vi "Day 2 task 2.vi"() -> ()   [LabVIEW 2022 SP3]
uses:
  <vilib>/regexp/Match Regular Expression.xnode
panel:
  out "sum":i32
  out "Array":i32[](array[numeric])
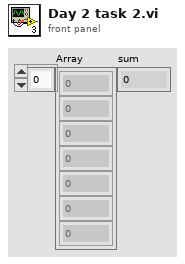
[diagram p1: front panel]
types:
  T1 = cluster{"Their":string, "Win":string, "Loose":string}[]
  T2 = cluster{"Mine":string, "Theirs":string, "Score":i32}[]
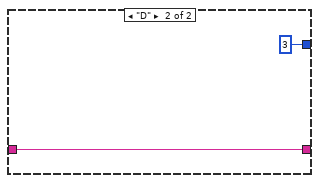
[diagram p2: hidden frame]
diagram:
  (unwired) "A Y\nB X\nC Z"
  (unwired) T2 [{"Mine"="R", "Theirs"="P", "Score"=0}, {"Mine"="R", "Theirs"="S", "Score"=6}, {"Mine"="P", "Theirs"="R", "Score"=6}, {"Mine"="P", "Theirs"="S", "Score"=0}, {"Mine"="S", "Theirs"="R", "Score"=0}, {"Mine"="S", "Theirs"="P", "Score"=6}]
  w9 = TRUE ("replace all? (F)")
  n1 = Search and Replace String(replace all?=w9, input string="C Y\nC Y\nB Y\nA Z\nB Z\nA X\nA Y\nA Y\nA X\nA Y\nB Y\nA Y\nB Y\nB Y\nB Z\nB Z\nB Z\nB Z\nA Y\nB Z\nA Y\nB X\nB Y\nB X\nA X\nA X\nB Z\nA X\nA X\nB Z\nB Z\nB Y\nB Z\nB Z\nB Z\nB Y\nA X\nA X\nB Z\nA X\nB X\nB X\nC Y\nB Z\nC X\nA X\nA Y\nB Y\nA Y\nB X\nA X\nB Y\nB Z\nB Z\nB Y\nB Z\nC Z\nB X\nB X\nB Z\nB Z\nB Z\nB Z\nA Y\nB X\nA X\nC X\nB Y\nB Z\nA Y\nB Z\nB Z\nB Y\nB Y\nB Z\nB Y\nB Z\nA X\nB X\nB X\nA X\nA X\nB Z\nB Z\nB Z\nB Z\nB Y\nB X\nB Z\nA X\nA Y\nB Z\nA Y\nB Z\nB Y\nB Z\nA X\nB Y\nA Y\nB Z\nA Z\nA Y\nA Y\nC Y\nB Z\nB X\nA Z\nB Z\nA X\nB Z\nA Z\nB Z\nA X\nB Y\nA X\nB Y\nB Z\nB X\nB X\nB Z\nB Z\nB Z\nA X\nB Z\nA X\nB X\nB Z\nA X\nC Z\nB Z\nB Z\nB Y\nB Y\nB Y\nB Z\nB Z\nA Y\nB Z\nB Z\nC Y\nC Z\nA X\nB Z\nB X\nB Z\nB Z\nB Y\nA X\nB Z\nB Y\nA Z\nB Z\nA X\nA X\nB Y\nA Y\nB Z\nB Z\nB X\nB Y\nA X\nA Y\nB X\nC Z\nA Y\nB Z\nB Z\nB Z\nA Z\nC Y\nB Y\nB Y\nB Z\nC Y\nB Y\nB X\nB X\nB Z\nC Z\nA X\nB Z\nB Z\nB Z\nB Z\nB X\nB X\nA X\nA Z\nA Z\nA X\nC Y\nB X\nA X\nA Y\nA X\nB X\nA Y\nB Z\nB Z\nA Y\nA X\nB Y\nB Z\nB Z\nA X\nA Z\nB Z\nB X\nA X\nB Z\nB Y\nA Y\nA Z\nB X\nA Y\nB Z\nA Z\nB Z\nA Y\nB Z\nB X\nB Y\nA Y\nB Z\nB Z\nA X\nA X\nB Y\nB Z\nA X\nB Z\nB Z\nB Z\nB Z\nB Z\nA Z\nB Z\nB Z\nB X\nA Y\nC X\nB Z\nB Y\nB Y\nB Z\nB Z\nB Z\nB Y\nB X\nB Y\nC X\nB Z\nA Z\nA Y\nC X\nA X\nB X\nA X\nB X\nA Y\nB Z\nA Y\nA Y\nB Z\nB X\nB Z\nA Y\nB Z\nB X\nC Z\nC X\nC Z\nB Y\nB X\nB Z\nB Z\nB Y\nB Z\nB Y\nB Z\nA X\nB X\nB Z\nA X\nB Z\nB Y\nB Z\nA X\nB Y\nC Y\nA Z\nB Z\nC Z\nA Y\nB Z\nA Y\nA Z\nB Y\nA X\nA X\nB Z\nB Z\nB Z\nA Y\nB Z\nA Z\nB Z\nA Y\nA Z\nB Y\nC Z\nB Z\nA Z\nB X\nB Z\nB Y\nB Z\nA Z\nA Z\nB Z\nB X\nC Z\nB X\nB Z\nB Y\nA X\nB Z\nA X\nB X\nB Z\nB Z\nA X\nB X\nC X\nC X\nB X\nB Y\nB Z\nB X\nB Y\nB Y\nB Z\nA Z\nB Z\nC X\nA Y\nC X\nB Z\nA Y\nB Z\nB Y\nB Z\nB X\nA X\nB X\nB Z\nA Y\nA Y\nB Z\nB Z\nB Z\nA Y\nB Z\nB X\nC X\nB Z\nB Z\nC Y\nB Z\nC Y\nB Z\nC Y\nC X\nB Z\nC Y\nA Y\nA Y\nC Z\nB Z\nB X\nB Z\nB X\nC Z\nB Z\nA Z\nB Z\nC Y\nB Z\nA X\nA Y\nB Y\nB Y\nB Z\nA Y\nB X\nB Z\nB Z\nA Z\nB X\nA Y\nA Y\nB Z\nB Z\nB Z\nC X\nA Z\nB X\nC Z\nB Y\nB Z\nB X\nA Y\nB Z\nA X\nB X\nB Y\nA Y\nB Z\nB Z\nB Y\nA Z\nB Z\nA X\nB Y\nA Y\nA X\nA Y\nA X\nA X\nB X\nB Y\nB X\nB Y\nB Z\nB Y\nB X\nA X\nB Z\nA Z\nA X\nB Z\nB Y\nA X\nB Y\nA X\nB X\nC Y\nB X\nB X\nB X\nC Y\nB X\nB Y\nB Y\nB Y\nB Y\nB X\nA Y\nC Y\nB Z\nB Z\nB X\nB Z\nC Y\nB Y\nB Z\nB Z\nB Y\nB Z\nA X\nB X\nB Y\nA X\nC Y\nB Z\nA Y\nB Z\nB Z\nB Z\nA X\nB Y\nB Z\nB Y\nB Z\nA X\nB Z\nA X\nB Y\nB Y\nB X\nB X\nA Y\nB Z\nC Y\nA X\nA X\nB X\nB Z\nB X\nB X\nB Z\nB Z\nA X\nB X\nB Z\nA Z\nB Y\nA X\nB Z\nC Y\nB Z\nB X\nB Z\nB Z\nA Y\nA Y\nB Z\nB X\nB Y\nB Z\nA Y\nA Y\nB X\nB X\nC X\nB Z\nC Z\nB X\nA Y\nB Z\nA Z\nB Y\nA Y\nB Z\nB X\nB X\nA Y\nB Z\nB Y\nA X\nB Y\nB Y\nB Y\nB X\nB Y\nB Z\nB Y\nB Y\nA X\nC Z\nB Z\nB Z\nA Z\nB Z\nB Z\nA X\nB X\nA Y\nA X\nB X\nC X\nB X\nB Z\nB Y\nA Z\nA Y\nB Y\nB Z\nB X\nB X\nB Z\nB Z\nB Y\nA X\nB Z\nA Y\nA X\nB Y\nB Z\nB Z\nB X\nA X\nA Y\nC X\nA Y\nB Z\nB Y\nB Z\nB Z\nC Z\nB Z\nB X\nA X\nC Y\nB X\nB Z\nA Z\nA X\nA Y\nB Z\nB Z\nA Y\nA Y\nB X\nA Y\nA Y\nB Z\nA Y\nB Y\nB Z\nA Y\nA Z\nB X\nB X\nB Y\nB Z\nB Z\nA X\nB X\nC X\nB Y\nA Y\nA X\nA X\nA X\nB Y\nA X\nA Z\nA Y\nB X\nA Y\nB Z\nC X\nB X\nB X\nB Z\nB X\nB X\nB Z\nA X\nB Z\nB X\nB Z\nA Y\nB Y\nB Z\nB Y\nB Z\nB Z\nA X\nB Z\nA Y\nC Z\nA Y\nB Z\nA Y\nB X\nB Z\nB X\nC Y\nA X\nB Z\nB Y\nA X\nA X\nB X\nB Z\nA Z\nB Z\nB X\nB X\nB X\nB Z\nB Z\nB Y\nB X\nB X\nA X\nB Z\nB X\nA X\nA X\nA X\nB X\nB Z\nA Z\nB X\nB Y\nB Y\nB Z\nB Z\nC Z\nA Y\nA X\nB Y\nB X\nB Z\nB X\nA X\nB Z\nB Z\nB Y\nB Z\nB X\nB Z\nB Z\nB X\nB X\nA X\nA X\nB X\nB Z\nB Z\nC X\nC X\nB Z\nB Z\nB X\nB Z\nB Y\nB X\nA X\nB Y\nA Y\nA X\nB Z\nB Z\nC X\nB Y\nB Z\nB Z\nB X\nB Z\nB Z\nC Z\nB Z\nB Y\nB Z\nB X\nA X\nB X\nB Z\nB Z\nA Y\nB Z\nB Z\nB Z\nB Z\nA X\nB Z\nB Z\nB X\nB Y\nB Y\nB Z\nA X\nB Z\nB Y\nB X\nA X\nB X\nB Z\nB Z\nB Z\nB X\nB Z\nB Z\nB Z\nA Y\nB Z\nC X\nB Y\nB Y\nB Y\nA Y\nB Z\nB Z\nA X\nC Z\nB Z\nB Z\nB Z\nB X\nB Z\nA Z\nB Z\nB Z\nB Z\nA Z\nB Z\nC Y\nB X\nA X\nA Y\nB Z\nB Z\nA Z\nB Z\nB X\nA Z\nB Y\nB Z\nB X\nB Z\nB X\nB Y\nB Z\nA X\nB Z\nB Z\nA Y\nB X\nB X\nB X\nA Z\nC X\nA Z\nB Z\nB Z\nB Z\nB X\nA Y\nC X\nA Z\nA Y\nB X\nB Z\nB X\nB Z\nB Y\nA Y\nB X\nC X\nA Y\nC Z\nA X\nB Z\nB Z\nA Z\nB X\nB Y\nB Z\nA Y\nB Y\nA X\nA X\nC Y\nA Y\nB X\nA X\nB Y\nB X\nB Y\nA Y\nA X\nC Y\nB Y\nB Y\nB Z\nB Y\nB X\nB Z\nB Z\nB X\nA X\nB Z\nB Z\nB Z\nB X\nB Z\nB X\nB Z\nB Z\nB Y\nB Y\nB X\nA X\nB Z\nB Y\nA Y\nB Z\nB X\nB Z\nB Z\nA Z\nB Z\nA Y\nB Z\nA X\nB Z\nB Z\nA Y\nB Z\nA X\nB Z\nA Y\nA Y\nA Z\nB X\nB Z\nB Y\nA Z\nC Z\nB Z\nA X\nA X\nB X\nA Z\nB X\nB X\nB Z\nC X\nB Z\nB Z\nB Z\nB Z\nB X\nA Z\nA Y\nB Z\nB Y\nC Z\nB Y\nB Z\nA Y\nB X\nB X\nB Z\nA X\nA Y\nB Z\nB X\nB Y\nA Y\nC Y\nC Y\nB Z\nA Y\nB Y\nA Y\nB Z\nB Z\nA X\nB X\nA X\nB X\nA Y\nA X\nB Z\nA X\nB Z\nB X\nB Z\nB X\nB X\nA X\nA Y\nB Z\nB X\nB X\nA X\nA Y\nA X\nB Y\nB Z\nB Z\nB Z\nB Z\nB Z\nB X\nB Y\nA Y\nB X\nB Z\nA Y\nB X\nA X\nB Z\nC X\nB Y\nA Y\nA X\nA X\nB X\nB X\nB Z\nB Z\nB Z\nB X\nB Y\nB X\nB Z\nB X\nB Y\nB X\nB Z\nB X\nB Y\nB X\nB Z\nB Z\nB Z\nA X\nC X\nC Y\nA Y\nB X\nB X\nA Y\nB Z\nB X\nB Z\nB X\nB X\nC X\nB Z\nB Z\nB Y\nA Z\nA Z\nC X\nB X\nC Y\nB Z\nC X\nB Z\nA Y\nC Z\nB X\nB Y\nA Y\nB Y\nB X\nB Z\nA Y\nA Z\nC X\nB Z\nA X\nB X\nB Z\nC Z\nA Y\nB Z\nB Z\nA X\nA X\nB Z\nB Y\nC Z\nB Z\nB X\nB Z\nA X\nA X\nB Y\nA X\nB X\nA Y\nB Z\nA Y\nB Z\nA Y\nB Z\nA X\nB Y\nB Z\nB Z\nB Z\nA X\nA X\nB X\nB Z\nA X\nB Z\nA X\nA X\nB Z\nB Z\nB Z\nB X\nB Y\nB Z\nB Z\nB X\nB Z\nB Y\nB Z\nC Y\nB X\nC Z\nB Z\nB Z\nA Y\nB Z\nB X\nA Y\nB Z\nB X\nB Z\nB Z\nB Y\nB Z\nA Z\nA Y\nB Z\nB Z\nB Y\nA Y\nB Z\nA X\nB X\nA Z\nA X\nB X\nB Z\nB X\nB Z\nB Z\nB Y\nB Y\nB Z\nB Y\nB Z\nB Z\nA X\nB X\nB Y\nB Y\nC Z\nA X\nB Y\nA Y\nB Z\nB Z\nB Z\nC X\nB X\nA Z\nB Y\nA X\nC X\nB Z\nB Z\nB Z\nB Y\nA Y\nA Y\nB Y\nB Z\nB Z\nB Z\nC X\nA X\nB Z\nA Y\nB X\nB Z\nB Z\nB Z\nB Z\nB X\nB Y\nB Z\nB Z\nA Y\nC X\nA X\nB Z\nB Z\nA Y\nA Y\nB Z\nA Y\nB Y\nA X\nB Z\nB Z\nA Y\nB Z\nB Z\nA X\nA X\nB X\nB Z\nB Z\nA X\nB Z\nB Z\nC Y\nB Z\nA X\nB Z\nA X\nB Z\nA X\nB X\nA X\nA Y\nB Z\nB X\nA X\nB Z\nA X\nA Z\nB Z\nB Z\nB Z\nA Y\nB X\nA X\nB Y\nA Y\nB Z\nB Z\nB X\nB Z\nB X\nB X\nA X\nB Z\nA Y\nA X\nB X\nA Z\nB X\nB Y\nB Z\nB X\nB X\nB Z\nC X\nA X\nB Z\nB Y\nC Z\nB Z\nA Z\nA Z\nA X\nA Y\nB Z\nB Z\nB X\nA Z\nB Z\nB Z\nB X\nB Y\nB X\nB Z\nB X\nB Z\nA Y\nA X\nB Z\nB X\nB Y\nB Z\nB Z\nB Z\nB Z\nC X\nC X\nB Z\nB X\nB Z\nB Z\nB Z\nB X\nB Z\nB Z\nB Z\nB X\nB Z\nB Z\nB Z\nC Y\nB Z\nB Y\nB Z\nA Z\nA Y\nB Z\nA Y\nC X\nA X\nB X\nA Y\nB Z\nA Y\nB Z\nB Y\nB Z\nB Z\nC Y\nB Y\nB Z\nB Z\nB X\nB Y\nB Z\nB Y\nB Z\nB X\nB Y\nB Z\nB Z\nB Z\nB Y\nB Y\nB Z\nB Z\nC X\nB Z\nA Y\nB Z\nB Z\nB Y\nB Y\nB Z\nB Z\nA Y\nB Z\nA Z\nC X\nA Y\nA Y\nA X\nB Z\nA X\nC Y\nA Z\nC Y\nC X\nB Z\nA X\nA Y\nB Z\nB Z\nB Z\nB Z\nB Y\nA Z\nA Y\nB Y\nA Y\nA Z\nB X\nB Z\nB Z\nA X\nC Y\nB Z\nB X\nC X\nA Z\nB Z\nB X\nB Y\nA X\nA X\nB Z\nC X\nB Z\nB Z\nB X\nB Z\nB Z\nB Z\nA X\nB Z\nB Y\nB Z\nB Z\nB Y\nB X\nA X\nB Z\nA X\nA X\nB Y\nB Z\nB X\nA Y\nC X\nB Y\nA X\nA X\nA X\nC Y\nB X\nC Z\nA X\nB Z\nA Z\nB Z\nA X\nA Y\nB Z\nA X\nB X\nA Y\nA X\nA Y\nB X\nB Y\nB Z\nB Y\nC X\nC Y\nB Z\nB Y\nB Z\nA X\nC Z\nB Z\nA X\nB X\nA X\nB X\nB Z\nB X\nB Z\nB Z\nB Z\nA X\nA X\nB Z\nB X\nB Z\nB Z\nB Z\nA X\nB Z\nB X\nA X\nC Z\nA Y\nB Z\nA Y\nB Z\nB Z\nB Z\nC Z\nB Z\nB Z\nA X\nB X\nA X\nB X\nA X\nB Z\nB Z\nB X\nB Z\nA X\nA Y\nA Y\nA Y\nB Z\nB Z\nB Z\nB Z\nA X\nB Z\nB Z\nB Y\nB Z\nA Z\nB Z\nA Y\nB Y\nB Y\nC Y\nB X\nB Z\nB Y\nB Z\nB Y\nB Z\nB Z\nA Y\nB X\nA Z\nB Z\nA X\nB Y\nA X\nB Z\nB Y\nA X\nB X\nB Z\nB Z\nB Z\nA Y\nA Y\nA X\nA Y\nA Y\nB X\nB Z\nB Y\nB Y\nB X\nB Y\nB X\nB X\nB X\nB Z\nB Z\nB Z\nA Y\nA Z\nB Y\nC X\nB X\nB Z\nC Y\nB Z\nC Y\nB Z\nB Z\nB Z\nB X\nA X\nB Z\nB Z\nA X\nB Z\nB Z\nB Z\nB Z\nB Z\nB Z\nB X\nA X\nA Y\nB Y\nB Z\nB Y\nB X\nA Z\nA X\nB X\nB Y\nB Z\nB Z\nB Z\nB X\nC X\nB X\nA Z\nA X\nA Y\nB Z\nB Z\nA X\nB Z\nA Y\nB X\nB Z\nB Y\nB Y\nA X\nB X\nB Z\nB Z\nB Z\nB Z\nB Y\nA Z\nA Y\nB X\nA X\nB Y\nB Z\nC Y\nB Z\nB Z\nB X\nA Z\nA Y\nB Y\nB Z\nA Y\nB Y\nA Y\nA X\nA Y\nB Y\nC X\nC Z\nB X\nA Z\nA X\nB Y\nB X\nA X\nB Z\nA Y\nA Z\nB Z\nB Z\nB Z\nA X\nB Z\nB Y\nB Z\nA X\nA Y\nB Z\nB X\nC X\nB Z\nA Y\nB Z\nB Z\nB X\nB Z\nB Z\nA Y\nA X\nB Z\nC Y\nA Y\nB Y\nB Z\nA X\nB Z\nB Z\nB Z\nB Z\nC X\nB Y\nB Z\nB X\nB Z\nB Z\nB Z\nB Z\nB Z\nB Y\nA X\nB Y\nA Y\nA X\nA X\nB Z\nB Z\nB Z\nC X\nB X\nB Z\nA X\nA X\nB Y\nA X\nB Z\nB Z\nB X\nB Y\nB Y\nB Y\nA Y\nA Y\nA X\nA X\nB Z\nB Y\nB Y\nB X\nB Y\nB Z\nA Z\nB Z\nA Z\nB X\nB Y\nC Y\nB X\nB X\nA X\nA X\nA X\nA X\nB Z\nB Z\nA Z\nB X\nB X\nB X\nB X\nB X\nB Z\nB Z\nB Z\nB Z\nB Z\nB Y\nB Z\nB Z\nA Y\nA Z\nC Y\nB Y\nA X\nB Z\nB X\nA Y\nB Y\nA Y\nC Z\nA X\nA Y\nB X\nB X\nC Z\nB Y\nA Y\nA Y\nA X\nB X\nA X\nB X\nA Y\nB Z\nB Z\nA Z\nB X\nB Z\nB Z\nB Y\nA Y\nB Z\nB Y\nB Z\nB Z\nB Z\nC X\nB Y\nA Y\nB Z\nA Y\nA Y\nA X\nB X\nB Y\nC Y\nC X\nB Z\nB Z\nB Z\nA Y\nA Z\nB Y\nB X\nB X\nB Y\nB Z\nB Z\nA Y\nB Y\nB Z\nB Z\nB Z\nA X\nC Y\nB Z\nA Z\nC Z\nB X\nB Y\nB Z\nA Z\nA X\nB X\nA X\nC X\nB Z\nA X\nB Y\nC Y\nB Y\nB Z\nB X\nA Y\nB Z\nB Z\nB Z\nA X\nB Z\nB Z\nB Z\nB Z\nA X\nB Z\nB X\nB X\nB Z\nC X\nA Y\nB Z\nB X\nB Z\nB Y\nB Z\nB Y\nC Y\nA X\nB Y\nB Z\nB Z\nB X\nB Z\nA X\nB Z\nA X\nB Y\nB Z\nA X\nB Z\nB X\nA Z\nB Z\nC X\nB Z\nB Y\nB Y\nB Y\nB Z\nB X\nB X\nA X\nA X\nB Z\nB Z\nA X\nA X\nA Z\nA Y\nC Z\nB Z\nB Y\nC X\nB X\nB Y\nB Y\nA Y\nB Z\nB Z\nB Y\nC Y\nB Z\nA Y\nB Z\nB Z\nB Z\nB Z\nA Y\nB Z\nB Z\nB Z\nA X\nB X\nA Y\nB Y\nB Z\nB Z\nB Z\nA Y\nB Z\nB Z\nB Z\nB Y\nB Y\nB X\nB X\nB Y\nC Z\nB X\nB Y\nC Y\nA Y\nB Z\nA Z\nB Z\nA Y\nB X\nB Z\nB X\nC Z\nA Y\nB X\nB Z\nA X\nA X\nB Z\nB Z\nB Y\nB Z\nC Y\nC X\nB Z\nB Z\nA X\nB X\nA Y\nB Y\nB Y\nC Z\nA X\nB X\nB Z\nA Y\nB Z\nC X\nB Z\nA Z\nC X\nA Y\nA Z\nB Z\nA Y\nA X\nB Z\nB Y\nB Z\nB X\nB Z\nA X\nB Z\nA Z\nB Z\nB Z\nB Y\nA X\nB Z\nB X\nB Y\nB Y\nA Y\nA X\nC Z\nB Y\nC Z\nA X\nB X\nB Z\nB X\nC X\nB Z\nB Z\nA X\nA Y\nA Z\nA Z\nB Z\nB Z\nA X\nB Z\nB Y\nA X\nA Y\nB Z\nB X\nA Y\nB Z\nB Y\nB X\nB Z\nA Z\nB Y\nA Y\nA X\nB Z\nB Z\nB Z\nB Z\nA X\nB Y\nB Z\nB Z\nB Z\nA Z\nB Y\nA X\nC Y\nB Z\nB Z\nB Y\nB X\nB Z\nA Y\nA X\nB Z\nB Y\nB Z\nA Y\nC X\nB Y\nB Z\nB Z\nA Y\nB X\nB Z\nB Z\nA X\nB X\nB Z\nA Z\nB Y\nB Z\nB Z\nB Z\nB Z\nB Z\nA Z\nB X\nA Y\nC Y\nB Z\nA Y\nB Z\nB Z\nA Y\nB Z\nB Z\nA Y\nA Y\nB X\nB Y\nA X\nB Z\nA Y\nB Z\nA Z\nB Z\nB X\nB Z\nB Z\nB Y\nB Y\nB Z\nA X\nB Y\nB Z\nB Z\nB Z\nB Y\nA Y\nB Z\nB Y\nB Z\nB Z\nB X\nA X\nB Y\nA X\nA X\nB Z\nA X\nB Z\nC X\nB Y\nB Z\nB Z\nB Y\nA X\nB Z\nB Z\nB Y\nB X\nB Z\nB X\nB Z\nC Y\nB Y\nB Z\nB Z\nA Z\nB Z\nB Z\nA Y\nB Z\nB Y\nA X\nB Z\nB Z\nB Z\nB X\nB Z\nB Y\nB Z\nB X\nC Z\nB Y\nB Z\nB Z\nB Y\nA X\nA X\nB Y\nA Y\nB Z\nB X\nB Y\nB Z\nB Y\nB Z\nA X\nC X\nB Z\nA Z\nC Y\nA X\nB Y\nB Y\nA X\nA X\nB Y\nB Z\nC Y\nB Z\nB Y\nA X\nB Y\nB Y\nB Z\nB X\nB Z\nC X\nC Y\nB X\nA Y\nB Z\nB Z\nB Z\nA X\nB Z\nB Z\nB X\nB X\nB X\nB X\nB Y\nA Y\nB Z\nB Z\nB Z\nA Z\nB X\nB X\nB X\nB X\nB Z\nA Y\nB Y\nB Z\nA X\nA X\nA X\nB Y\nB Z\nB X\nB Z\nA Z\nB Z\nB Z\nA Y\nC Z\nA X\nB Z\nC X\nB Z\nB Z\nB Z\nB Y\nB Y\nB Z\nC X\nB Z\nA Y\nB X\nC X\nA Y\nC X\nB Z\nB X\nA Z\nB Z\nC Y\nB Y\nB X\nB Z\nB Y\nA Y\nB X\nA Z\nB Z\nB Z\nC Z\nB Z\nB Y\nB Z\nA Y\nC Y\nB Z\nB X\nA Y\nB Z\nB Z\nB Y\nB Y\nB Z\nA X\nA Y\nA X\nA Z\nB Z\nB Z\nB Y\nA Y\nB Y\nB Z\nB Y\nA Y\nB X\nA X\nB Y\nB Y\nB X\nB Z\nB Y\nC X\nB Z\nB Z\nB Z\nA X\nB Z\nB X\nA Y\nA Y\nB Z\nA Y\nA Y\nA Y\nB Y\nB Z\nA X\nC X\nB Y\nA X\nC X\nB Z\nB Y\nA Y\nB X\nB Z\nB Y\nB Y\nB Z\nB Z\nA Y\nB X\nB X\nA X\nB Z\nB X\nB Z\nB Z\nC Z\nC Y\nA X\nB X\nC X\nB X\nA Z\nA X\nB Y\nC X\nB Y\nA X\nA X\nA X\nB X\nB Z\nB X\nB Y\nB Z\nB Z\nB Z\nB Z\nA X\nA X\nB X\nB Z\nA Z\nA X\nB Z\nC Y\nB Z\nA X\nB Z\nA Z\nB Z\nB Z\nA Y\nB Y\nB Z\nB X\nB Z\nB Z\nC Y\nB Z\nB X\nA X\nB Y\nB Z\nA Y\nA X\nB Z\nB Y\nB Z\nB X\nA Y\nC Z\nB X\nB Z\nA X\nB X\nB Z\nB Z\nA X\nB Y\nB X\nB Z\nB Z\nB Y\nB X\nB X\nC X\nB Z\nC X\nB Z\nC Y\nA Y\nC X\nB X\nB Y\nB Z\nB Y\nB Z\nA X\nB Z\nB Z\nB Y\nB Y\nA X\nA X\nA Y\nB Z\nB Z\nA Y\nB Z\nA X\nB Z\nB X\nB X\nB X\nA Y\nB Z\nB Z\nA Y\nB Z\nA Z\nB Y\nB X\nA Z\nA Z\nB Z\nA Y\nB Z\nB Y\nB Y\nB X\nA Y\nB X\nB Z\nB Z\nB Y\nB X\nB Z\nB Z\nB Z\nB Z\nA X\nB X\nB X\nB Z\nA X\nB X\nB Z\nB Z\nB Y\nA Y\nB Z\nB Y\nB Y\nA X\nB X\nB Y\nC X\nC X\nB Y\nA Y\nA Z\nB X\nB Z\nB Z\nB Z\nB Z\nA X\nA Y\nA Y\nB Y\nC X\nB Z\nA Y\nB X\nC Z\nB X\nB Y\nA Y\nB X\nB Y\nB Z\nB Y\nB X\nB Y\nA Z\nB Z\nA X\nB X\nB X\nB Z\nB Y\nB Y\nB Y\nA X\nB X\nB Y\nB Z\nA Y\nA X\nB X\nB Z\nB Z\nC X\nA Z\nB Z\nA X\nA Y\nC X\nB Z\nB Z\nA X\nB X\nA Y\nA Y\nB Z\nB Z\nB X\nA Z\nB Z\nB Y\nA Y\nB Z\nB Y\nA Y\nB Y\nB Z\nA X\nB Y\nA X\nA Y\nA X\nA X\nB Y\nA Z\nB Z\nA Y\nB Z\nA Z\nA Y\nB Z\nB Y\nB Z\nB X", search string="A", replace string="R" ("replace string (\"\")"), error in=errorcluster {"status"=FALSE, "code"=0, "source"=""}) -> (result string=w27:string, error out=w21:errorcluster)  [unwired: 3 in, 2 out]
  n2 = Search and Replace String(replace all?=w9, input string=w27, search string="B", replace string="P" ("replace string (\"\")"), error in=w21) -> (result string=w23:string, error out=w20:errorcluster)  [unwired: 3 in, 2 out]
  n3 = Search and Replace String(replace all?=w9, input string=w23, search string="C", replace string="S" ("replace string (\"\")"), error in=w20) -> (result string=w7:string, error out=w8:errorcluster)  [unwired: 3 in, 2 out]
  n4 = Search and Replace String(replace all?=w9, input string=w7, search string="X", replace string="L" ("replace string (\"\")"), error in=w8) -> (result string=w12:string, error out=w18:errorcluster)  [unwired: 3 in, 2 out]
  n5 = Search and Replace String(replace all?=w9, input string=w12, search string="Y", replace string="D" ("replace string (\"\")"), error in=w18) -> (result string=w16:string, error out=w19:errorcluster)  [unwired: 3 in, 2 out]
  n6 = Search and Replace String(replace all?=w9, input string=w16, search string="Z", replace string="W" ("replace string (\"\")"), error in=w19) -> (result string=w6:string, error out=w5:errorcluster)  [unwired: 3 in, 2 out]
  n7 = Spreadsheet String To Array(delimiter (Tab)="\n", format string="%s", spreadsheet string=w6, array type (2D Dbl)=string[] []) -> (array=w31:string[])
  n8 = for {
    tunnel: w31 -> [w46] mode=indexing
    tunnel: w5 -> [w45]
    tunnel: cluster{"Mine":string, "Score":i32}[] [{"Mine"="R", "Score"=1}, {"Mine"="P", "Score"=2}, {"Mine"="S", "Score"=3}] -> [w43]
    tunnel: [w42] -> w3 mode=indexing
    tunnel: T1 [{"Their"="R", "Win"="P", "Loose"="S"}, {"Their"="P", "Win"="S", "Loose"="R"}, {"Their"="S", "Win"="R", "Loose"="P"}] -> [w36]
    n9 = xnode "Match Regular Expression"("input string"=w46, "regular expression"="\\s", "error in"=w45) -> ("before match"=w39:string, "after match"=w40:string)  [unwired: 3 in, 3 out]
    n10 = case shown="\"W\", Default" w40 {
      selector: w40 -> [w55 _]
      tunnel: w39 -> [w56 w65]
      tunnel: [w51 w65] -> w38
      tunnel: [w49 3] -> w37
      tunnel: w36 -> [w57 _]
      frame "W", Default {
        n11 = for {
          tunnel: w57 -> [w63] mode=indexing
          tunnel: [w62] -> w52
          tunnel: [w61] -> w53
          tunnel: w56 -> [w59]
          stop <- w58 stop-if-true
          n12 = Unbundle By Name(w63) -> ("Their"=w60:string, "Win"=w62:string, "Loose"=w61:string)
          n13 = Equal?(x=w59, y=w60) -> (x = y?=w58:bool)
        }
        n14 = Equal?(x="W", y=w55) -> (x = y?=w50:bool)
        n15 = Select(t=6, s=w50, f=0) -> (s? t:f=w49:i32)
        n16 = Select(t=w52, s=w50, f=w53) -> (s? t:f=w51:string)
      }
      frame "D" {
      }
    }
    n17 = for {
      tunnel: w43 -> [w70] mode=indexing
      tunnel: [w67] -> w41
      tunnel: w38 -> [w66]
      stop <- w68 stop-if-true
      n18 = Unbundle(w70) -> ("Mine"=w69:string, "Score"=w67:i32)
      n19 = Equal?(x=w66, y=w69) -> (x = y?=w68:bool)
    }
    n20 = Add(x=w37, y=w41) -> (x+y=w42:i32)
  }
  "Array" <- w3
  n21 = Add Array Elements(numeric array=w3) -> (sum=→"sum":i32)
